vi "VIve LabVIEW_MAIN_Menu.vi"(0 "Buttons name":T2={"Caption.button0"="Starts the test sequence", "Button.name0"="Measure", "Caption.button1"="Cross correlation", "Button.name1"="Analyze", "Caption.button2"="Prints the test data report", "Button.name2"="Present", "Caption.button3"="Quits the application", "Button.name3"="Exit"}, 9 "Colors":T1={"False state Button color"=16118498, "True state  Button color"=10983021, "Focused color"=12826781, "Decoration Color"=2098432}) -> (6 "Button number":i32=1, 8 "Boton.name selected":string="Measure", 15 "error out":errorcluster)   [LabVIEW 2009]
panel:
  in  "Button4":bool
  in  "Button3":bool
  in  "Button2":bool
  in  "Button1":bool
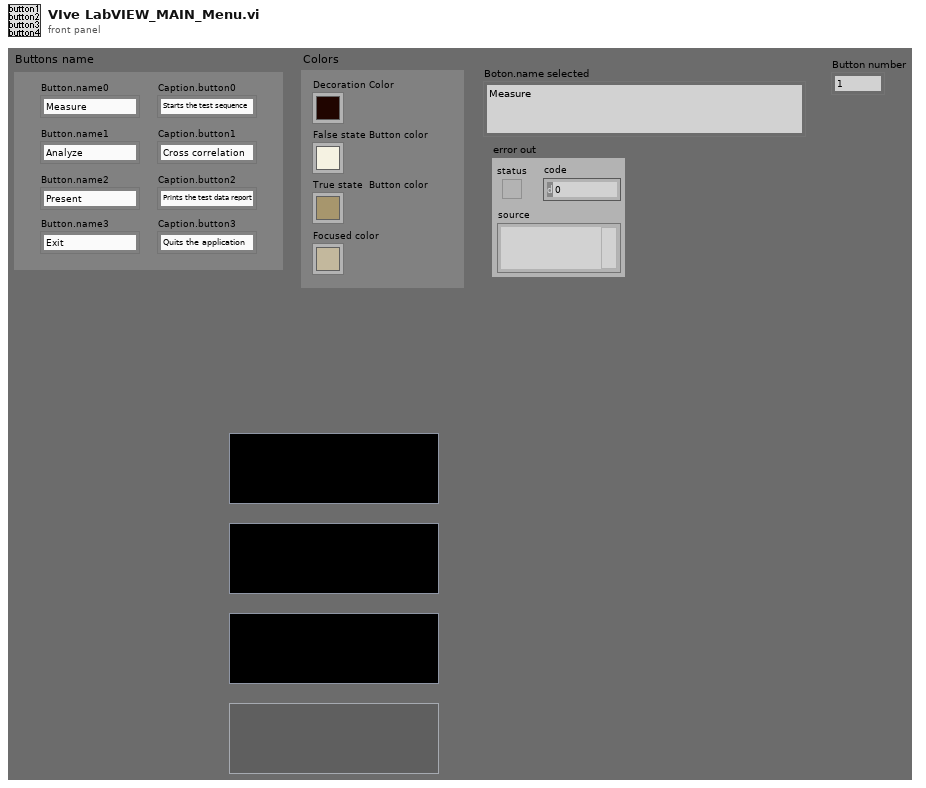
[diagram p1: front panel]
types:
  T1 = cluster{"False state Button color":u32, "True state  Button color":u32, "Focused color":u32, "Decoration Color":u32}
  T2 = cluster{"Caption.button0":string, "Button.name0":string, "Caption.button1":string, "Button.name1":string, "Caption.button2":string, "Button.name2":string, "Caption.button3":string, "Button.name3":string}
  T3 = typedef "lveventtype.ctl" = enum32{"Null", "Timeout", "App Instance Close", "App Instance Close?", "Cell Edit", "Cell Edit?", "Cursor Grab", "Cursor Grab?", "Cursor Move", "Cursor Release", "Data Change", "Direction Change", "Display State Change", "Drag Ended", "Drag Enter", "Drag Leave", "Drag Over", "Drag Source Update", "Drag Starting", "Drag Starting?", "Drop", "Exec State Change", "Key Down", "Key Down?", "Key Repeat", "Key Repeat?", "Key Up", "Listbox Double Click", "Menu Activation?", "Menu Selection (App)", "Menu Selection? (App)", "Menu Selection (User)", "Mouse Down", "Mouse Down?", "Mouse Enter", "Mouse Leave", "Mouse Move", "Mouse Up", "NI Security User Change (App)", "Pane Size", "Panel Close", "Panel Close?", "Panel Resize", "Plot Attribute Change", "Scale Range Change", "Shortcut Menu Activation?", "Shortcut Menu Selection (App)", "Shortcut Menu Selection? (App)", "Shortcut Menu Selection (User)", "Tree Double Click", "Tree Drag", "Tree Drag?", "Tree Drop", "Tree Drop?", "Tree Item Close", "Tree Item Close?", "Tree Item Open", "Tree Item Open?", "Value Change"}
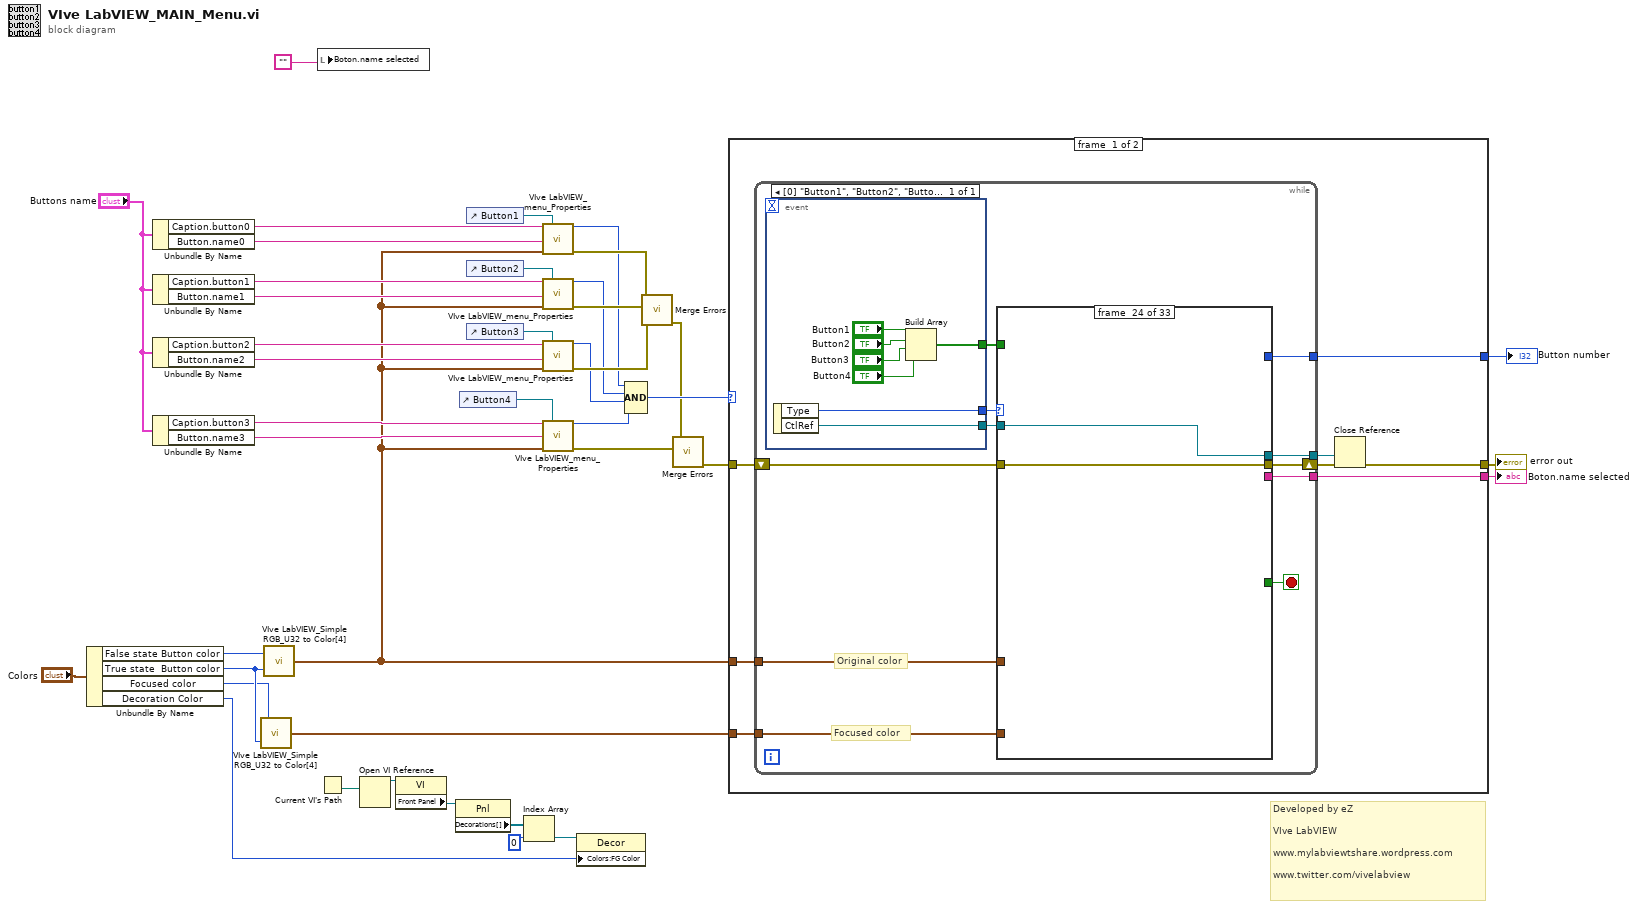
[diagram p0: block diagram]
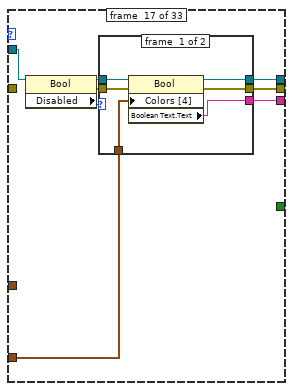
[diagram p18: hidden frame]
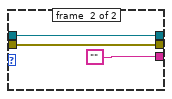
[diagram p19: hidden frame]
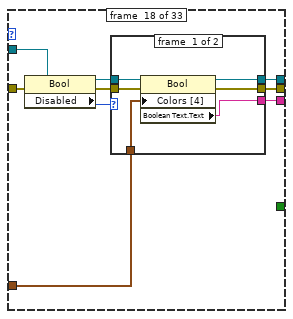
[diagram p20: hidden frame]
diagram:
  # "Developed by eZ\n\nVIve LabVIEW\n\nwww.mylabviewtshare.wordpress.com\n\nwww.twitter.com/vivelabview"
  n1 = Unbundle By Name("Colors") -> ("False state Button color"=w32:u32, "True state  Button color"=w34:u32, "Focused color"=w33:u32, "Decoration Color"=w25:u32)
  n2 = Unbundle By Name("Buttons name") -> ("Caption.button0"=w19:string, "Button.name0"=w18:string)
  n3 = Unbundle By Name("Buttons name") -> ("Caption.button1"=w17:string, "Button.name1"=w16:string)
  n4 = Unbundle By Name("Buttons name") -> ("Caption.button2"=w13:string, "Button.name2"=w12:string)
  n5 = Unbundle By Name("Buttons name") -> ("Caption.button3"=w10:string, "Button.name3"=w11:string)
  n6 = call "VIve LabVIEW_Simple RGB_U32 to Color[4].vi"("False state  RGB_U32 2"=w34, "True state RGB_U32"=w33) -> ("Colors[4]"=w41:cluster{u32, u32}[])  [unwired: 1 in]
  n7 = call "VIve LabVIEW_Simple RGB_U32 to Color[4].vi"("False state  RGB_U32 2"=w34, "True state RGB_U32"=w32) -> ("Colors[4]"=w9:cluster{u32, u32}[])  [unwired: 1 in]
  n8 = local write "Boton.name selected"("") -> ()
  n9 = Current VI's Path() -> (path=w31:path)
  n10 = Open VI Reference(vi path=w31) -> (vi reference=w30:refnum<vi>)  [unwired: 5 in, 1 out]
  n11 = property class="VI"(reference=w30) -> ("Front Panel"=w29:refnum<vi>)  [unwired: 1 in, 2 out]
  n12 = property class="Pnl"(reference=w29) -> ("Decorations[]"=w28:refnum<vi>[])  [unwired: 1 in, 2 out]
  n13 = control-ref of="Button4"() -> (w1:refnum<vi>)
  n14 = control-ref of="Button1"() -> (w20:refnum<vi>)
  n15 = control-ref of="Button2"() -> (w15:refnum<vi>)
  n16 = control-ref of="Button3"() -> (w14:refnum<vi>)
  n17 = Index Array(array=w28, index=0) -> (element=w26:refnum<vi>)
  n18 = call "VIve LabVIEW_menu_Properties.vi"("Caption.button"=w19, "reference"=w20, "Button.name"=w18, "Colors[4]"=w9) -> ("Disabled"=w2:u8, "error out"=w22:errorcluster)  [unwired: 10 in]
  n19 = call "VIve LabVIEW_menu_Properties.vi"("Caption.button"=w17, "reference"=w15, "Button.name"=w16, "Colors[4]"=w9) -> ("Disabled"=w3:u8, "error out"=w21:errorcluster)  [unwired: 10 in]
  n20 = call "VIve LabVIEW_menu_Properties.vi"("Caption.button"=w13, "reference"=w14, "Button.name"=w12, "Colors[4]"=w9) -> ("Disabled"=w4:u8, "error out"=w8:errorcluster)  [unwired: 10 in]
  n21 = call "VIve LabVIEW_menu_Properties.vi"("Caption.button"=w10, "reference"=w1, "Button.name"=w11, "Colors[4]"=w9) -> ("Disabled"=w5:u8, "error out"=w7:errorcluster)  [unwired: 10 in]
  n22 = property class="Decor"(reference=w26, "Colors:FG Color"=w25) -> ()  [unwired: 1 in, 2 out]
  n23 = Compound Arithmetic op=AND(w2, w3, w4, w5) -> (w39:u8)
  n24 = call <vilib>:"Merge Errors.vi"("error in 3 (no error)"=w8, "error in 2 (no error)"=w21, "error in 1 (no error)"=w22) -> ("error out"=w37:errorcluster)  [unwired: 4 in]
  n25 = call <vilib>:"Merge Errors.vi"("error in 2 (no error)"=w7, "error in 1 (no error)"=w37) -> ("error out"=w36:errorcluster)  [unwired: 5 in]
  n26 = case shown="0" w39 {
    tunnel: w9 -> [w49 _]
    tunnel: w41 -> [w48 _]
    tunnel: [w44 w178] -> w38
    tunnel: w36 -> [w46 w179]
    tunnel: [w43 ""] -> w23
    tunnel: [w42 -1] -> w24
    frame #0 {
      n27 = while {
        tunnel: [w59] -> w43
        tunnel: [w56] -> w47
        tunnel: w49 -> [w54]
        tunnel: w48 -> [w55]
        shift-right: [w53] -> w45
        shift-left: w46 -> [w52]
        tunnel: [w50] -> w42
        stop <- w58 stop-if-true
        # "Focused color"
        # "Original color"
        n28 = event shown="[0] \"Button1\", \"Button2\", \"Button3\", \"Button4\": Value Change;  \"Button1\", \"Button2\", \"Button3\", \"Button4\": Mouse Enter;  \"Button1\", \"Button2\", \"Button3\", \"Button4\": Mouse Leave" {
          selector: _ -> [_]
          dyn-events: _ -> [_]
          timeout: _ -> [_]
          tunnel: [w171] -> w60
          tunnel: [w172] -> w57
          tunnel: [w166] -> w51
          event [0] "Button1", "Button2", "Button3", "Button4": Value Change;  "Button1", "Button2", "Button3", "Button4": Mouse Enter;  "Button1", "Button2", "Button3", "Button4": Mouse Leave {
            n29 = event-data() -> ("Type"=w171:T3, "CtlRef"=w172:refnum<vi>)  [unwired: 1 in]
            n30 = Build Array("Button1", "Button2", "Button3", "Button4") -> (w166:bool[])
          }
        }
        n31 = case shown="\"Value Change\"" w60 {
          tunnel: [_ _ _ _ _ _ _ _ _ _ _ _ _ _ _ _ w93 w115 _ _ _ _ _ _ _ _ _ _ _ _ _ _ w164] -> w59
          tunnel: [_ _ _ _ _ _ _ _ _ _ _ _ _ _ _ _ _ _ _ _ _ _ _ _ _ _ _ _ _ _ _ _ TRUE] -> w58
          tunnel: w57 -> [w62 w64 w66 w68 w70 w72 w74 w76 w78 w80 w82 w84 w86 w88 w90 w92 w97 w114 w129 w131 w133 w135 w137 w139 w141 w143 w145 w147 w149 w151 w153 w155 w163]
          tunnel: [w62 w64 w66 w68 w70 w72 w74 w76 w78 w80 w82 w84 w86 w88 w90 w92 w95 w118 w129 w131 w133 w135 w137 w139 w141 w143 w145 w147 w149 w151 w153 w155 w162] -> w56
          tunnel: w55 -> [_ _ _ _ _ _ _ _ _ _ _ _ _ _ _ _ w96 _ _ _ _ _ _ _ _ _ _ _ _ _ _ _ _]
          tunnel: w54 -> [_ _ _ _ _ _ _ _ _ _ _ _ _ _ _ _ _ w117 _ _ _ _ _ _ _ _ _ _ _ _ _ _ w161]
          tunnel: [w61 w63 w65 w67 w69 w71 w73 w75 w77 w79 w81 w83 w85 w87 w89 w91 w94 w116 w128 w130 w132 w134 w136 w138 w140 w142 w144 w146 w148 w150 w152 w154 w160] -> w53
          tunnel: w52 -> [w61 w63 w65 w67 w69 w71 w73 w75 w77 w79 w81 w83 w85 w87 w89 w91 _ w110 w128 w130 w132 w134 w136 w138 w140 w142 w144 w146 w148 w150 w152 w154 w159]
          tunnel: w51 -> [_ _ _ _ _ _ _ _ _ _ _ _ _ _ _ _ _ _ _ _ _ _ _ _ _ _ _ _ _ _ _ _ w158]
          tunnel: [_ _ _ _ _ _ _ _ _ _ _ _ _ _ _ _ _ _ _ _ _ _ _ _ _ _ _ _ _ _ _ _ w156] -> w50
          frame #0 {
          }
          frame #1 {
          }
          frame #2 {
          }
          frame #3 {
          }
          frame #4 {
          }
          frame #5 {
          }
          frame #6 {
          }
          frame #7 {
          }
          frame #8 {
          }
          frame #9 {
          }
          frame #10 {
          }
          frame #11 {
          }
          frame #12 {
          }
          frame #13 {
          }
          frame #14 {
          }
          frame #15 {
          }
          frame #16 {
            n32 = property class="Bool"(reference=w97) -> (reference out=w99:refnum<vi>, error out=w98:errorcluster, "Disabled"=w100:u8)  [unwired: 1 in]
            n33 = case shown="0" w100 {
              tunnel: [w106 w109] -> w95
              tunnel: w96 -> [w105 _]
              tunnel: [w104 w107] -> w94
              tunnel: [w103 ""] -> w93
              tunnel: w99 -> [w102 w109]
              tunnel: w98 -> [w101 w107]
              frame #0 {
                n34 = property class="Bool"(reference=w102, error in=w101, "Colors [4]"=w105) -> (reference out=w106:refnum<vi>, error out=w104:errorcluster, "Boolean Text.Text"=w103:string)
              }
              frame #1 {
              }
            }
          }
          frame #17 {
            n35 = property class="Bool"(reference=w114, error in=w110) -> (reference out=w112:refnum<vi>, error out=w111:errorcluster, "Disabled"=w113:u8)
            n36 = case shown="0" w113 {
              tunnel: [w124 w127] -> w118
              tunnel: w117 -> [w123 _]
              tunnel: [w122 w125] -> w116
              tunnel: [w121 ""] -> w115
              tunnel: w112 -> [w120 w127]
              tunnel: w111 -> [w119 w125]
              frame #0 {
                n37 = property class="Bool"(reference=w120, error in=w119, "Colors [4]"=w123) -> (reference out=w124:refnum<vi>, error out=w122:errorcluster, "Boolean Text.Text"=w121:string)
              }
              frame #1 {
              }
            }
          }
          frame #18 {
          }
          frame #19 {
          }
          frame #20 {
          }
          frame #21 {
          }
          frame #22 {
          }
          frame #23 {
          }
          frame #24 {
          }
          frame #25 {
          }
          frame #26 {
          }
          frame #27 {
          }
          frame #28 {
          }
          frame #29 {
          }
          frame #30 {
          }
          frame #31 {
          }
          frame #32 {
            n38 = property class="Bool"(reference=w163, error in=w159, "Colors [4]"=w161) -> (reference out=w162:refnum<vi>, error out=w160:errorcluster, "Boolean Text.Text"=w164:string)
            n39 = Search 1D Array(1D array=w158, element=TRUE) -> (index of element=w156:i32)  [unwired: 1 in]
          }
        }
      }
      n40 = Close Reference(reference=w47, error in (no error)=w45) -> (error out=w44:errorcluster)
    }
    frame #1 {
      n41 = Bundle By Name(cluster=w179, "status"=TRUE, "code"=5000, "source"="Error: All buttons are disabled") -> (w178:errorcluster)
    }
  }
  "error out" <- w38
  "Boton.name selected" <- w23
  "Button number" <- w24
